vi "CS SQL Server.Global.vi"(1 "command":T1(ring)=enum."default", 4 "connection":refnum<k5>) -> (18 "Open Connections":refnum<k5>[](array[refnum]))   [LabVIEW 2014, in "CS SQL Server.lvlib"]
doc: "THis FGV is used to maintain the list of open connections."
uses:
  CS SQL Server.lvlib
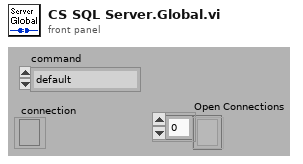
[diagram p1: front panel]
types:
  T1 = enum16{"add connection", "remove connection", "kill all connections", "default"}
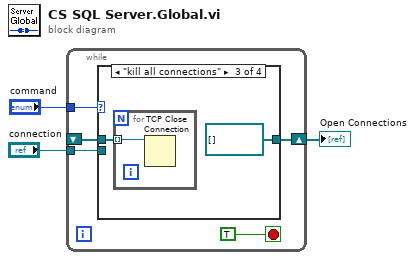
[diagram p0: block diagram]
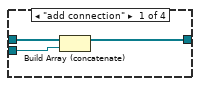
[diagram p2: hidden frame]
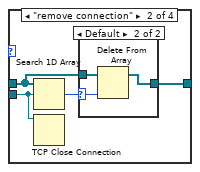
[diagram p3: hidden frame]
diagram:
  n1 = while {
    shift-right: [w8] -> w1
    shift-left: _ -> [w7]
    tunnel: "command" -> [w5]
    tunnel: "connection" -> [w4]
    stop <- TRUE stop-if-true
    n2 = case shown="\"kill all connections\"" w5 {
      tunnel: w7 -> [w11 w15 w20 w23]
      tunnel: [w9 w14 refnum<k5>[] [] w23] -> w8
      tunnel: w4 -> [w10 w12 _ _]
      frame "add connection" {
        n3 = Build Array (concatenate)(w11, w10) -> (w9:refnum<k5>[])
      }
      frame "remove connection" {
        n4 = Search 1D Array(1D array=w15, element=w12) -> (index of element=w13:i32)  [unwired: 1 in]
        n5 = TCP Close Connection(connection ID=w12) -> ()  [unwired: 2 in, 2 out]
        n6 = case shown="Default" w13 {
          selector: w13 -> [_ w17]
          tunnel: w15 -> [w16 w19]
          tunnel: [w16 w18] -> w14
          frame -1 {
          }
          frame Default {
            n7 = Delete From Array(array=w19, index=w17) -> (array with subset deleted=w18:refnum<k5>[])  [unwired: 1 in, 1 out]
          }
        }
      }
      frame "kill all connections" {
        n8 = for {
          tunnel: w20 -> [w22] mode=indexing
          n9 = TCP Close Connection(connection ID=w22) -> ()  [unwired: 2 in, 2 out]
        }
      }
      frame Default {
      }
    }
  }
  "Open Connections" <- w1
